vi "Update time chart -- subVI.vi"(8 "error in (no error)":errorcluster, 9 "Val read":dbl, 10 "Initial time":u32, 11 "Time chart in":cluster{"Angle":dbl, "Data":dbl}[](array[cluster])) -> (0 "error out":errorcluster, 3 "Time chart out":cluster{"Time":dbl, "Data":dbl}[](array[cluster]))   [LabVIEW 2020]
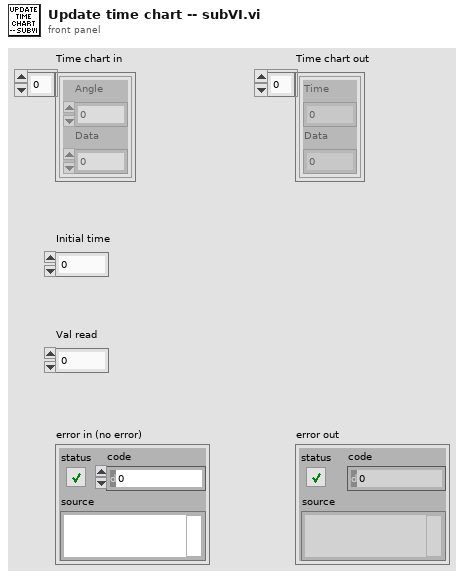
[diagram p1: front panel]
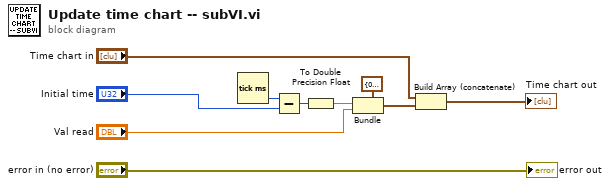
[diagram p0: block diagram]
diagram:
  n1 = Tick Count (ms)() -> (millisecond timer value=w3:u32)
  n2 = Subtract(x=w3, y="Initial time") -> (x-y=w5:u32)
  n3 = To Double Precision Float(number=w5) -> (double precision float=w6:dbl)
  n4 = Bundle(cluster=cluster{"Time":dbl, "Data":dbl} {"Time"=0.0, "Data"=0.0} ("Time chart"), "Time"=w6, "Data"="Val read") -> (w8:cluster{"Time":dbl, "Data":dbl})
  n5 = Build Array (concatenate)("Time chart in", w8) -> (→"Time chart out":cluster{"Time":dbl, "Data":dbl}[])
  "error out" <- "error in (no error)"
